vi "RunAudioProcPython.vi"() -> ()   [LabVIEW 2017]
panel:
  out "array":dbl[](array[numeric])
  out "standard error":string
  out "standard output":string
  in  "working directory":path=path ""
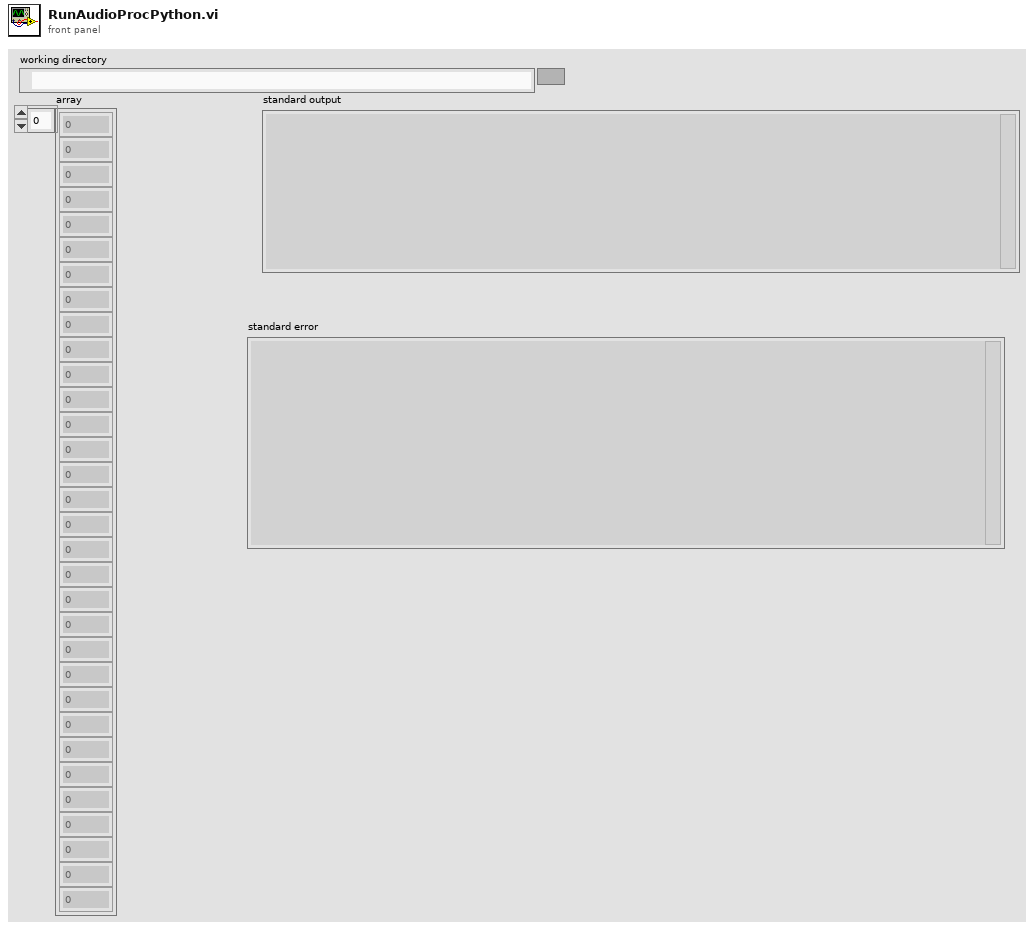
[diagram p1: front panel]
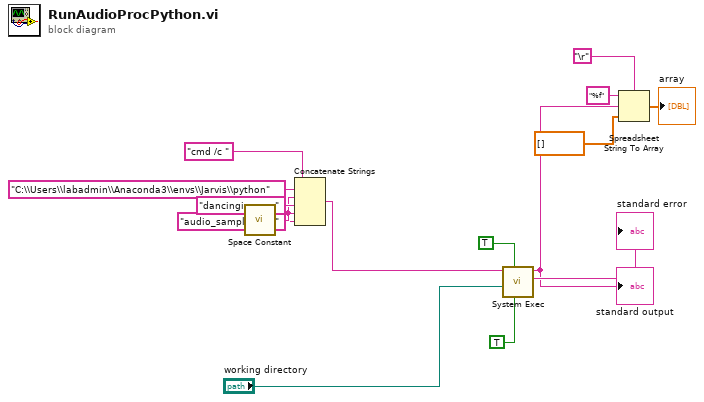
[diagram p0: block diagram]
diagram:
  n1 = call <vilib>:"Space Constant.vi"() -> ("String"=w9:string)
  n2 = Concatenate Strings("cmd /c " ("string"), "C:\\Users\\labadmin\\Anaconda3\\envs\\Jarvis\\python" ("string"), w9, "dancingions.py" ("string"), w9, "audio_sample.mp3" ("string")) -> (w7:string)
  n3 = call <vilib>:"System Exec.vi"("run minimized? (F)"=TRUE, "wait until completion? (T)"=TRUE, "working directory"="working directory", "command line"=w7) -> ("standard error"=→"standard error":string, "standard output"=w5:string)  [unwired: 4 in, 2 out]
  "standard output" <- w5
  n4 = Spreadsheet String To Array(delimiter (Tab)="\r", format string="%f", spreadsheet string=w5, array type (2D Dbl)=dbl[] []) -> (array=→"array":dbl[])
